vi "Configure Individual Limit Test.vi"(0 "VISA resource name":refnum<visa-resource-name>, 1 "Limit Test Upper Limit (1)":dbl=1.0, 2 "Enable Limit Test (F: Disable)":bool, 3 "Limit Test Type (1: Limit)":i32(ring)=1 items=["Compliance", "Limit"], 5 "Channel (0: Channel 1)":i32(ring) items=["Channel 1", "Channel 2"], 7 "Limit Test Number (1)":i32=1, 11 "error in (no error)":errorcluster, 12 "Limit Test Lower Limit (-1)":dbl=-1.0, 13 "Compliance Test Judgement Criteria (0: In)":i32(ring) items=["In", "Out"]) -> (4 "VISA resource name out":refnum<visa-resource-name>, 15 "error out":errorcluster)   [LabVIEW 2023, in "Agilent B2900 Series.lvlib"]
doc: "Configures the properties of specified limit test. The limit test means a pass/fail judgement performed while a composite limit test. The limit test result is returned by Read Limit Test Result.vi \n\n<B>Note:</B>\nThis VI is not applicable for Agilent models B2961A, B2962A, B2961B, B2962B, B2961C and B2962C."
uses:
  Agilent B2900 Series.lvlib
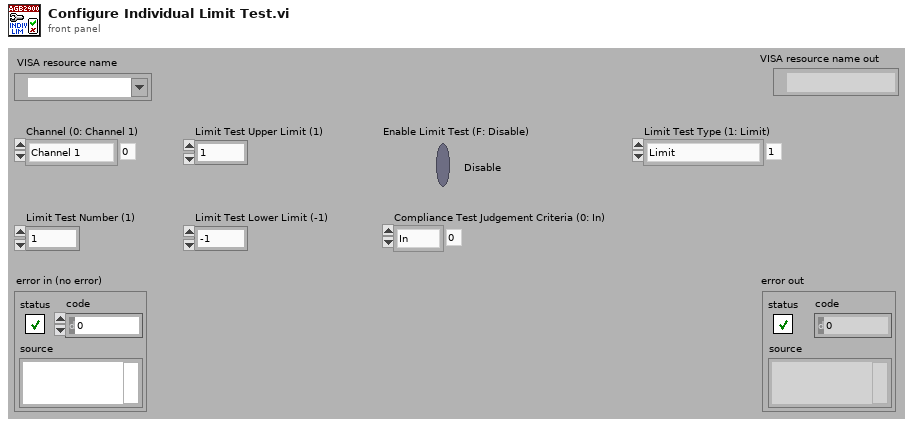
[diagram p1: front panel]
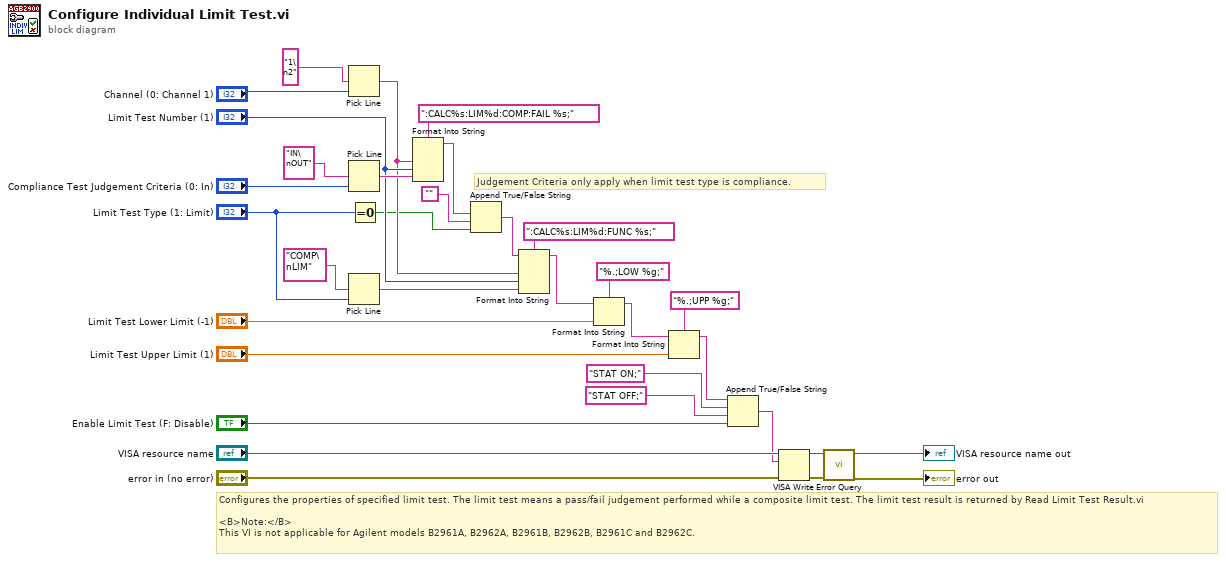
[diagram p0: block diagram]
diagram:
  # "Configures the properties of specified limit test. The limit test means a pass/fail judgement performed while a composite limit test. The limit test result is returned by Read Limit Test Result.vi \n\n<B>Note:</B>\nThis VI is not applicable for Agilent models B2961A, B2962A, B2961B, B2962B, B2961C and B2962C."
  # "Judgement Criteria only apply when limit test type is compliance."
  n1 = Pick Line(multi-line string="1\n2" ("string (\"\")"), line index="Channel (0: Channel 1)") -> (output string=w6:string)  [unwired: 1 in]
  n2 = Pick Line(multi-line string="IN\nOUT", line index="Compliance Test Judgement Criteria (0: In)") -> (output string=w9:string)  [unwired: 1 in]
  n3 = Pick Line(multi-line string="COMP\nLIM", line index="Limit Test Type (1: Limit)") -> (output string=w7:string)  [unwired: 1 in]
  n4 = Equal To 0?(x="Limit Test Type (1: Limit)") -> (x = 0?=w2:bool)
  n5 = Format Into String(format string=":CALC%s:LIM%d:COMP:FAIL %s;", w6, "Limit Test Number (1)", w9) -> (resulting string=w4:string)  [unwired: 2 in, 1 out]
  n6 = Append True/False String(1:w2, 2:"", 3:w4) -> (0:w12:string)  [unwired: 1 in]
  n7 = Format Into String(format string=":CALC%s:LIM%d:FUNC %s;", initial string=w12, w6, "Limit Test Number (1)", w7) -> (resulting string=w31:string)  [unwired: 1 in, 1 out]
  n8 = Format Into String(format string="%.;LOW %g;", initial string=w31, "Limit Test Lower Limit (-1)") -> (resulting string=w28:string)  [unwired: 1 in, 1 out]
  n9 = Format Into String(format string="%.;UPP %g;", initial string=w28, "Limit Test Upper Limit (1)") -> (resulting string=w25:string)  [unwired: 1 in, 1 out]
  n10 = Append True/False String(1:"Enable Limit Test (F: Disable)", 2:"STAT OFF;", 3:"STAT ON;", 4:w25) -> (0:w5:string)
  n11 = VISA Write(VISA resource name="VISA resource name", write buffer=w5, error in (no error)="error in (no error)") -> (VISA resource name out=w19:refnum<visa-resource-name>, error out=w18:errorcluster)  [unwired: 1 out]
  n12 = call "Error Query.vi"("error in (no error)"=w18, "VISA resource name"=w19) -> ("error out"=→"error out":errorcluster, "VISA resource name out"=→"VISA resource name out":refnum<visa-resource-name>)  [unwired: 6 in, 2 out]
